vi "LV2Climb.vi"(8 "error in (no error)":errorcluster, 11 "Elevator in":refnum<class "Elevator.lvclass">) -> (0 "error out":errorcluster, 3 "Elevator out":refnum<class "Elevator.lvclass">)   [LabVIEW 2019, in "Elevator.lvlib" / "Elevator.lvclass"]
uses:
  Elevator.lvclass
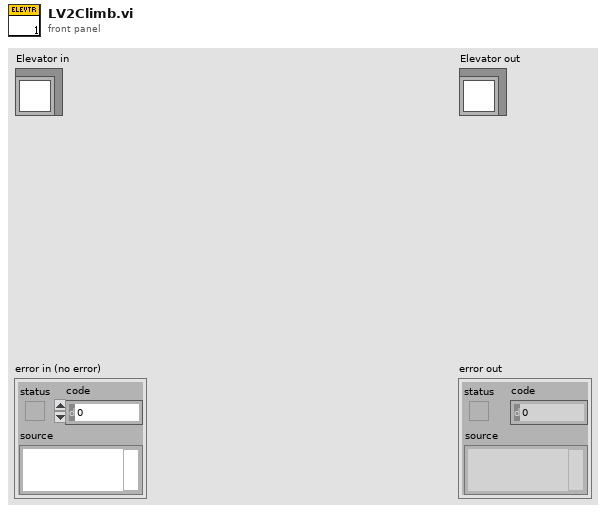
[diagram p1: front panel]
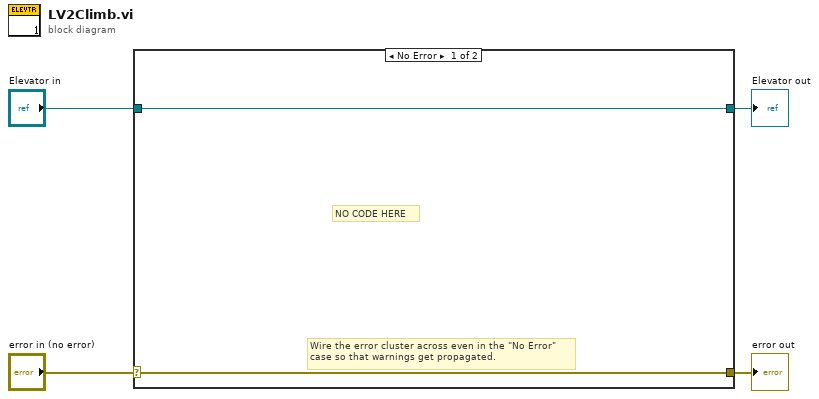
[diagram p0: block diagram]
diagram:
  n1 = case shown="No Error" "error in (no error)" {
    selector: "error in (no error)" -> [w5 w8]
    tunnel: [w5 w8] -> w3
    tunnel: [w6 w7] -> w1
    tunnel: "Elevator in" -> [w6 w7]
    frame No Error {
      # "NO CODE HERE"
      # "Wire the error cluster across even in the \"No Error\"\ncase so that warnings get propagated."
    }
    frame Error {
    }
  }
  "error out" <- w3
  "Elevator out" <- w1
